vi "End Undo.vi"(7 "Successful Operation ?":bool=TRUE, 8 "error in (no error)":errorcluster, 11 "Vi Ref":refnum<vi>) -> (0 "error out":errorcluster, 3 "Vi Ref Out":refnum<vi>)   [LabVIEW 2012, in "Scripting Tools.lvlib"]
doc: "Finishes the Undo transaction. If Successful Operation ? is true (default) the undo transaction completes and the changes are retained. If false, the transaction is rolled back."
uses:
  Scripting Tools.lvlib
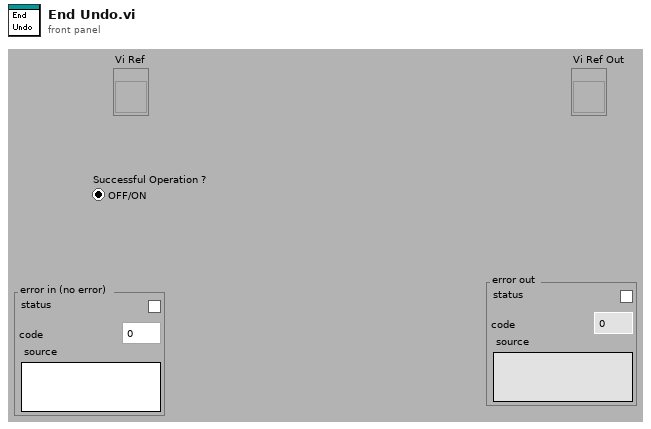
[diagram p1: front panel]
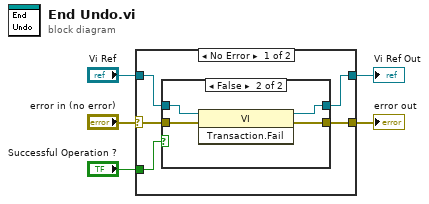
[diagram p0: block diagram]
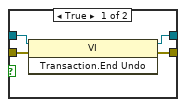
[diagram p2: hidden frame]
diagram:
  n1 = case shown="No Error" "error in (no error)" {
    selector: "error in (no error)" -> [w9 w20]
    tunnel: [w6 w20] -> w4
    tunnel: [w7 w19] -> w3
    tunnel: "Vi Ref" -> [w10 w19]
    tunnel: "Successful Operation ?" -> [w8 _]
    frame No Error {
      n2 = case shown="False" w8 {
        tunnel: w10 -> [w14 w18]
        tunnel: w9 -> [w13 w17]
        tunnel: [w12 w16] -> w7
        tunnel: [w11 w15] -> w6
        frame True {
          n3 = invoke class="VI" method="Transaction.End Undo"(reference=w14, error in=w13) -> (reference out=w12:refnum<vi>, error out=w11:errorcluster)  [unwired: 1 in, 1 out]
        }
        frame False {
          n4 = invoke class="VI" method="Transaction.Fail"(reference=w18, error in=w17) -> (reference out=w16:refnum<vi>, error out=w15:errorcluster)  [unwired: 1 in, 1 out]
        }
      }
    }
    frame Error {
    }
  }
  "error out" <- w4
  "Vi Ref Out" <- w3
